vi "Write to YAML File.vi"(8 "error in (no error)":errorcluster, 10 "Anything":variant, 11 "File Path":path) -> (0 "error out":errorcluster, 2 "YAML String":string, 3 "File Path out":path)   [LabVIEW 2015, in "YAML Parser.lvlib"]
uses:
  YAML Parser.lvlib
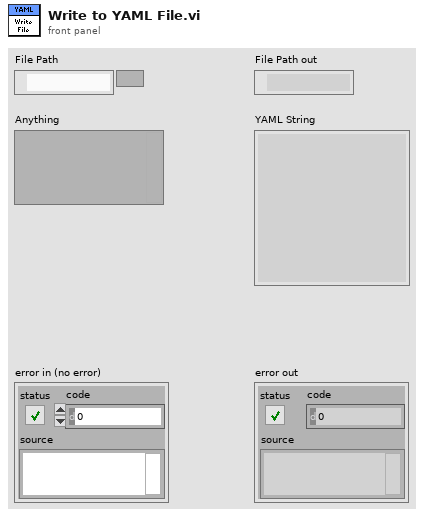
[diagram p1: front panel]
types:
  T1 = enum16{"open", "replace", "create", "open or create", "replace or create", "replace or create with confirmation"}
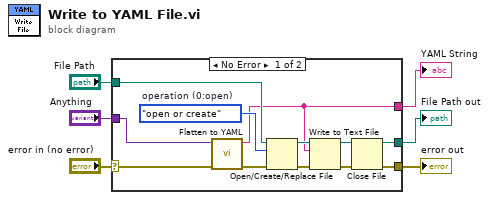
[diagram p0: block diagram]
diagram:
  n1 = case shown="No Error" "error in (no error)" {
    selector: "error in (no error)" -> [w17 w20]
    tunnel: "Anything" -> [w18 _]
    tunnel: [w9 w20] -> w5
    tunnel: [w7 _] -> w1
    tunnel: "File Path" -> [w11 w19]
    tunnel: [w10 w19] -> w2
    frame No Error {
      w8 = T1."open or create"  # operation (0:open)
      n2 = call "Flatten to YAML.vi"("error in (no error)"=w17, "Anything"=w18) -> ("error out"=w12:errorcluster, "YAML String"=w7:string)  [unwired: 8 in]
      n3 = Open/Create/Replace File(file path (use dialog)=w11, error in=w12, operation (0:open)=w8) -> (refnum out=w16:refnum<file>, error out=w15:errorcluster)  [unwired: 3 in, 1 out]
      n4 = Write to Text File(file (use dialog)=w16, text=w7, error in=w15) -> (refnum out=w14:refnum<file>, error out=w13:errorcluster)  [unwired: 1 in, 1 out]
      n5 = Close File(refnum=w14, error in=w13) -> (path=w10:path, error out=w9:errorcluster)
    }
    frame Error {
    }
  }
  "File Path out" <- w2
  "YAML String" <- w1
  "error out" <- w5
